vi "TelloDemoExample.vi"(9 "Command":T6, 10 "Tello IP":T5="192.168.1.10") -> (2 "Return":string)   [LabVIEW 2018]
uses:
  Library/Central Controller/TypeDef/TelloCommands.ctl
  Library/Central Controller/TypeDef/TelloIP.ctl
  Library/Central Controller/TypeDef/VideoOutState.ctl
  <vilib>/Platform/TimedLoop/XDataNode/timing_clust.ctl
  <vilib>/Platform/TimedLoop/XDataNode/nitl_modes.ctl
  <vilib>/Platform/TimedLoop/XDataNode/wakeup.ctl
  <vilib>/addons/control/pid/pid.llb/PID (DBL).vi
  <vilib>/Utility/inputDevices.llb/keyboardAcquire.vi
  <vilib>/Utility/inputDevices.llb/closeKeyboard.vi
  <vilib>/platform/TimedLoop/XDataNode/XDataNode.xnode
  Library/Simple UDP Message/Simple UDP Message.lvlib
  <vilib>/Platform/TimedLoop/XDataNode/XDNodeRunTimeDep.lvlib
  <vilib>/addons/control/pid/NI_PID_pid.lvlib
panel:
  out "IterationsPID":i64
  in  "Time switch back to frame from Tello":dbl=0.2 caption="Time Target (s)"
  in  "bkgY":i32=240
  out "VideoState":T1
  out "VideoOut":T2(plugin-control)
  out "Time has Elapsed":bool
  out "TellodetBallFalse":bool
  out "frameFromCam":T2(plugin-control)
  in  "Min Radius (Circle Detection 1) 2":sgl(slide)=9.0 scale=0.0..10.0
  in  "Max Radius (Circle Detection 1) 2":sgl(slide)=100.0 scale=10.0..50.0
  out "Nb Circles2":i32
  out "Circles Data (Circle Detection 1) 2":T3(array[cluster])
  out "Pos. X 2":i32
  in  "Red or Hue Range (Color Threshold 1) 2":cluster{"Lower value":i32, "Upper value":i32}={"Lower value"=20, "Upper value"=40}
  in  "Green or Sat Range (Color Threshold 1) 2":cluster{"Lower value":i32, "Upper value":i32}={"Lower value"=100, "Upper value"=250}
  in  "Blue or Luma or Val or Inten Range (Color Threshold 1) 2":cluster{"Lower value":i32, "Upper value":i32}={"Lower value"=98, "Upper value"=250}
  out "Pos. Y 2":i32
  in  "setpointY":dbl=150.0 format="%#_13g"
  in  "Up/Down PID":T4={"proportional gain (Kc)"=0.30000000000000004, "integral time (Ti, min)"=0.0, "derivative time (Td, min)"=0.001} {"derivative time (Td, min)" format="%.4f"; "integral time (Ti, min)" format="%.4f"; "proportional gain (Kc)" format="%.3f"}
  out "Pos. Y":i32
  in  "Blue or Luma or Val or Inten Range (Color Threshold 1)":cluster{"Lower value":i32, "Upper value":i32}={"Lower value"=98, "Upper value"=250}
  in  "Green or Sat Range (Color Threshold 1)":cluster{"Lower value":i32, "Upper value":i32}={"Lower value"=100, "Upper value"=250}
  in  "Red or Hue Range (Color Threshold 1)":cluster{"Lower value":i32, "Upper value":i32}={"Lower value"=20, "Upper value"=40}
  in  "Yaw PID":T4={"proportional gain (Kc)"=0.233, "integral time (Ti, min)"=0.0, "derivative time (Td, min)"=0.001} {"derivative time (Td, min)" format="%.4f"; "integral time (Ti, min)" format="%.4f"; "proportional gain (Kc)" format="%.3f"}
  out "Pos. X":i32
  in  "followBall":bool
  in  "Ball Detect":bool
  out "Circles Data (Circle Detection 1)":T3(array[cluster])
  out "Nb Circles1":i32
  in  "Max Radius (Circle Detection 1)":sgl(slide)=100.0 scale=10.0..50.0
  in  "Min Radius (Circle Detection 1)":sgl(slide)=9.0 scale=0.0..10.0
  out "frameFromTello":T2(plugin-control)
  out "Stop":bool
  out "RC command String":string
  in  "fly?":bool
  out "tilt l/r, f/b":cluster{dbl[], dbl[]}(graph)
  out "yaw, up/down":cluster{dbl[], dbl[]}(graph)
  out "rc command":string
  out "commands":i32
  out "restart":i32
  out "trials":i32
  in  "Send Cmd":bool
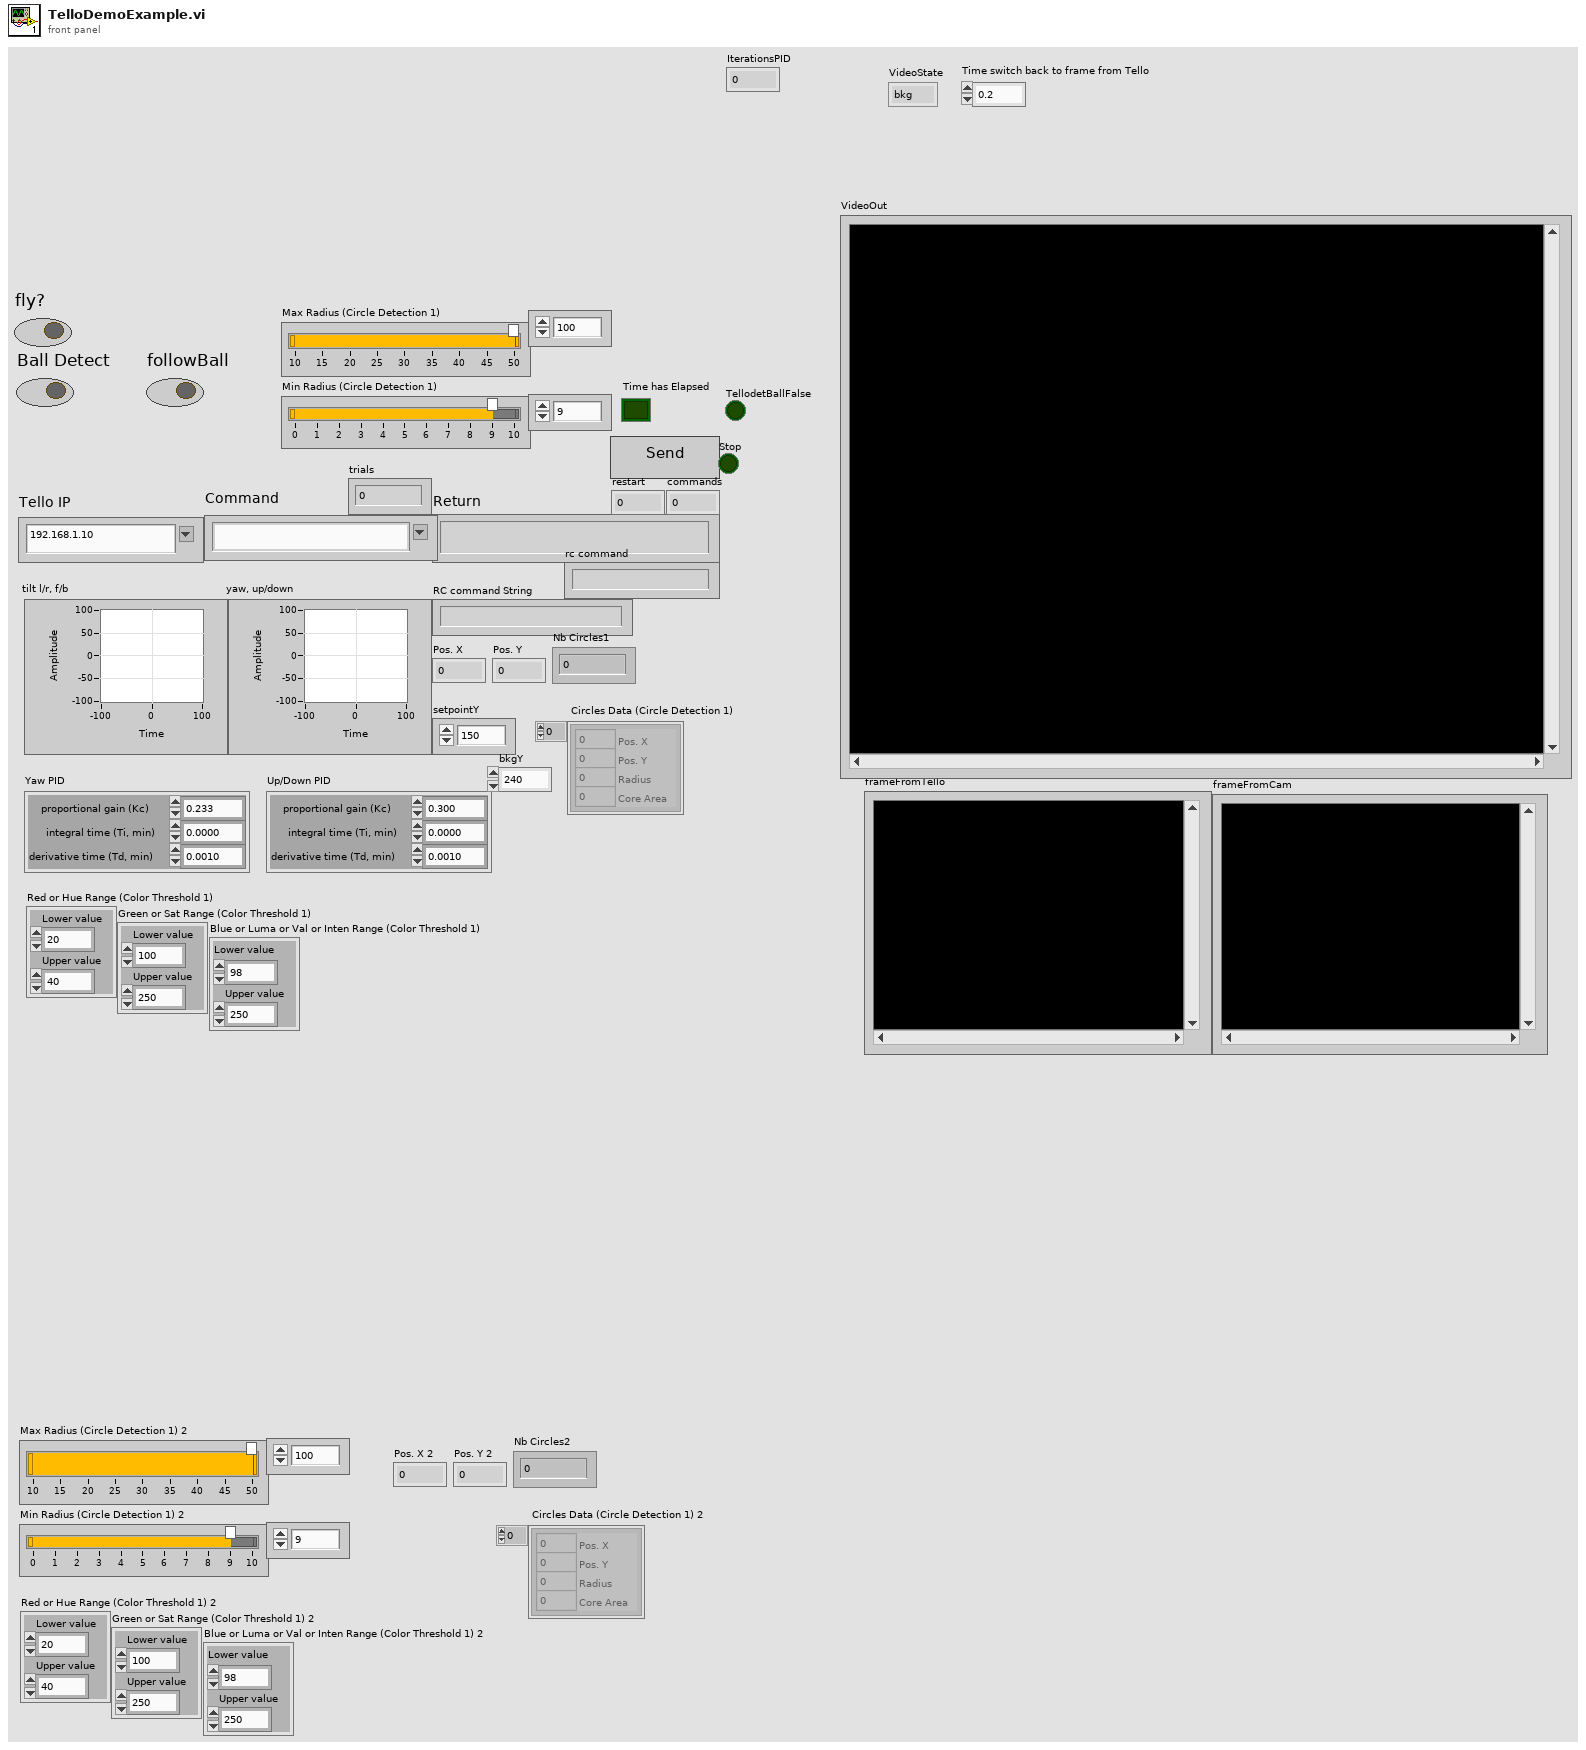
[diagram p1: front panel]
types:
  T1 = typedef "VideoOutState.ctl" = enum16{"bkg", "Tello"}
  T2 = typedef "IMAQ Image.ctl" = refnum<image>
  T3 = cluster{"Pos. X":i32, "Pos. Y":i32, "Radius":i32, "Core Area":i32}[]
  T4 = cluster{"proportional gain (Kc)":dbl, "integral time (Ti, min)":dbl, "derivative time (Td, min)":dbl}
  T5 = typedef "TelloIP.ctl" = string
  T6 = typedef "TelloCommands.ctl" = string
  T7 = typedef "Image Type" = u32
  T8 = typedef "XDNodeRunTimeDep.lvlib/timing_clust.ctl" = cluster{"Expected End [f-1]":u64, "Actual End [f-1]":u64, "Finished Late? [f-1]":bool, "Expected End [i-1]":u64, "Actual End [i-1]":u64, "Finished Late? [i-1]":bool, "Expected Start [i]":u64, "Actual Start [i]":u64, "Expected Start [f]":u64, "Actual Start [f]":u64, "Source Name":string, "Structure Name":string, "Period":i64, "Deadline":i64, "Offset":i64, "Start":i64, "Priority":i32, "Timeout":i32, "Mode":T9, "Wakeup Reason":T10, "Error":errorcluster, "Source Type":string, "Secondary Source Type":string, "Global End Time":u64, "Global Start Time":u64, "Frame Duration":u64, "Iteration Duration":u64, "Assigned CPU":i32, "I/O Scan Engine Mode":u32}
  T9 = typedef "XDNodeRunTimeDep.lvlib/nitl_modes.ctl" = enum32{"No Change", "Process missed periods, maintain original phase", "Discard missed periods, maintain original phase", "Process missed periods, ignore original phase", "Discard missed periods, ignore original phase"}
  T10 = typedef "XDNodeRunTimeDep.lvlib/wakeup.ctl" = enum32{"Normal", "Aborted", "Asynchronous wakeup", "Timing source error", "Timed loop error", "Timeout"}
  T11 = enum16{"0", "1", "2", "3", "4", "5", "6", "7", "8", "9", "A", "B", "C", "D", "E", "F", "G", "H", "I", "J", "K", "L", "M", "N", "O", "P", "Q", "R", "S", "T", "U", "V", "W", "X", "Y", "Z", "F1", "F2", "F3", "F4", "F5", "F6", "F7", "F8", "F9", "F10", "F11", "F12", "F13", "F14", "F15", "ADD", "BACK", "BACKSLASH", "CAPITAL", "COMMA", "DECIMAL", "DELETE", "DIVIDE", "DOWN", "END", "EQUALS", "ESCAPE", "GRAVE (`)", "HOME", "INSERT", "LBRACKET", "LCONTROL", "LEFT", "L ALT", "LSHIFT", "LWIN", "MINUS", "MULTIPLY", "NEXT", "NUMLOCK", "NUMPAD_0", "NUMPAD_1", "NUMPAD_2", "NUMPAD_3", "NUMPAD_4", "NUMPAD_5", "NUMPAD_6", "NUMPAD_7", "NUMPAD_8", "NUMPAD_9", "PAUSE", "PERIOD", "PRIOR (PG UP)", "RBRACKET", "RCONTROL", "RETURN", "RIGHT", "R ALT", "RSHIFT", "RWIN", "SCROLL", "SEMICOLON", "SLASH", "SPACE", "SUBTRACT", "TAB", "UP", "ENTER (num pad)", "' (quote)"}
  T12 = enum16{"0", "1", "2", "3", "4", "5", "6", "7", "8", "9", "A", "B", "C", "D", "E", "F", "G", "H", "I", "J", "K", "L", "M", "N", "O", "P", "Q", "R", "S", "T", "U", "V", "W", "X", "Y", "Z", "F1", "F2", "F3", "F4", "F5", "F6", "F7", "F8", "F9", "F10", "F11", "F12", "F13", "F14", "F15", "ADD", "BACK", "BACKSLASH", "CAPITAL", "COMMA", "DECIMAL", "DELETE", "DIVIDE", "DOWN", "END", "EQUALS", "ESCAPE", "GRAVE (`)", "HOME", "INSERT", "LBRACKET", "LCONTROL", "LEFT", "L ALT", "LSHIFT", "LWIN", "MINUS", "MULTIPLY", "NEXT", "NUMLOCK", "NUMPAD_0", "NUMPAD_1", "NUMPAD_2", "NUMPAD_3", "NUMPAD_4", "NUMPAD_5", "NUMPAD_6", "NUMPAD_7", "NUMPAD_8", "NUMPAD_9", "PAUSE", "PERIOD", "PRIOR (PG UP)", "RBRACKET", "RCONTROL", "RETURN", "RIGHT", "R ALT", "RSHIFT", "RWIN", "SCROLL", "SEMICOLON", "SLASH", "SPACE", "SUBTRACT", "TAB", "UP", "ENTER (num pad)", "' (quote)"}[]
  T13 = cluster{"Left":i32, "Top":i32, "Right":i32, "Bottom":i32}
  T14 = cluster{"Pos. X":i32, "Pos. Y":i32, "Radius":i32, "Core Area":i32}
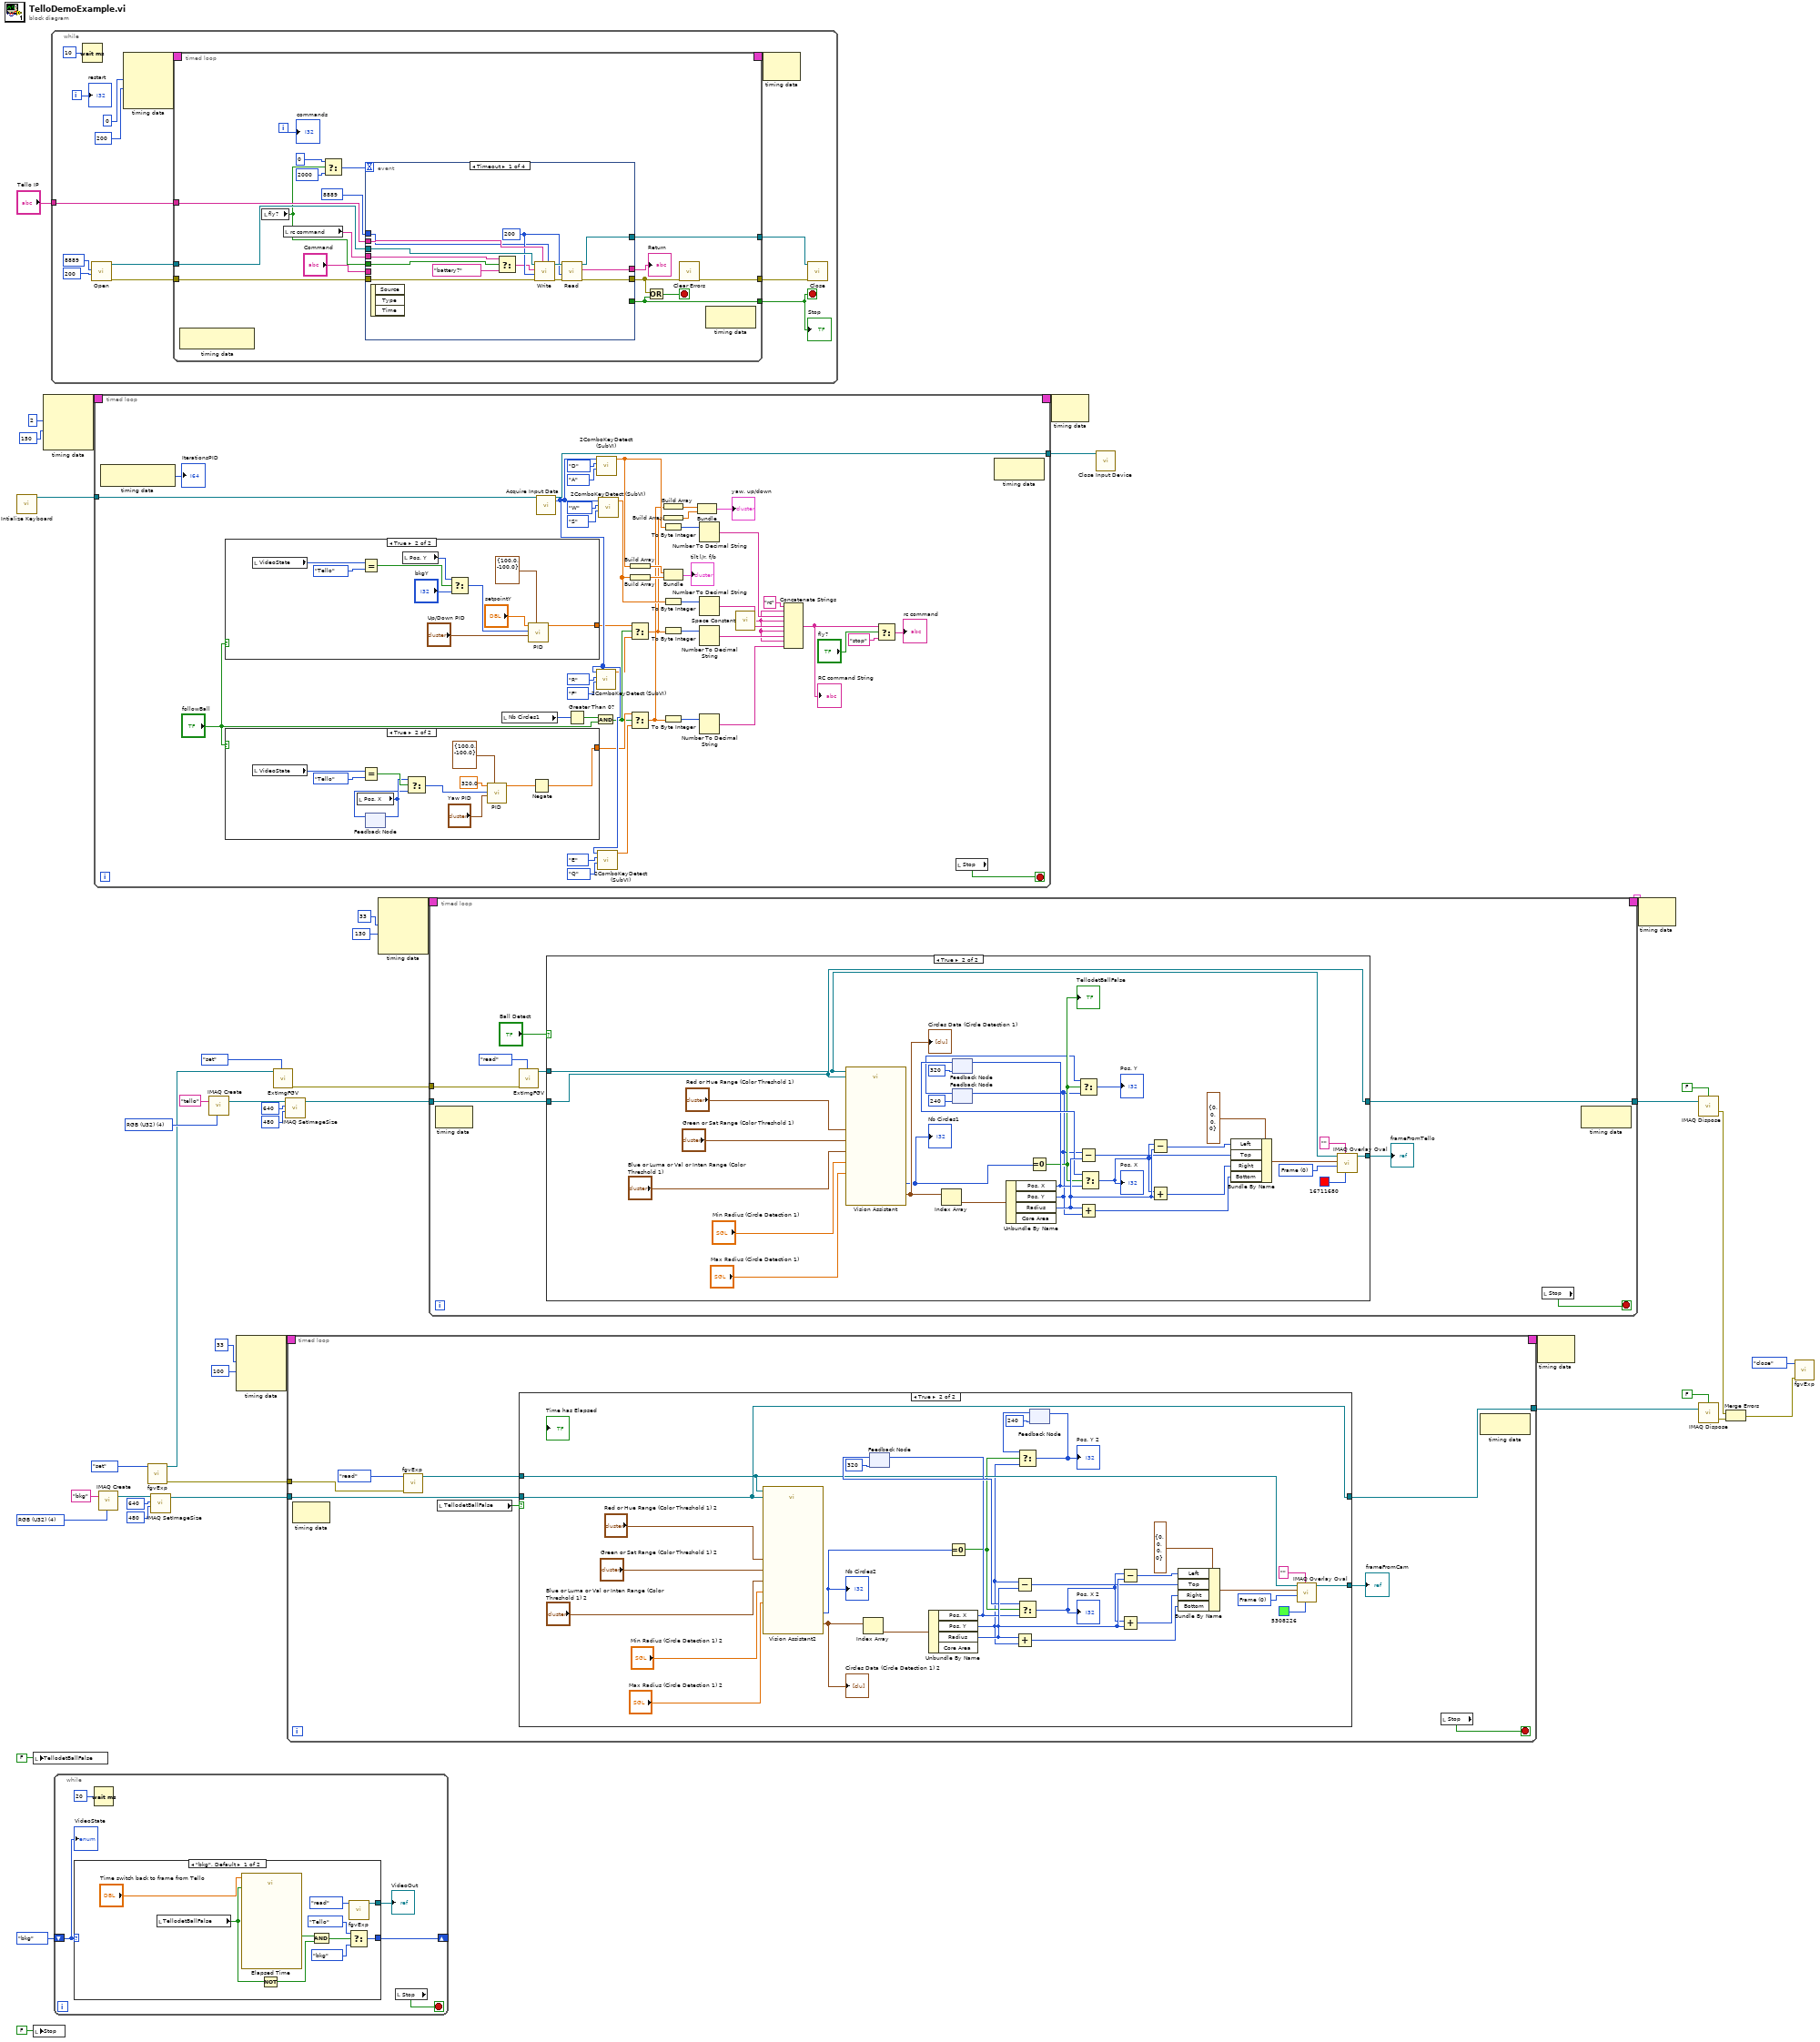
[diagram p0: block diagram]
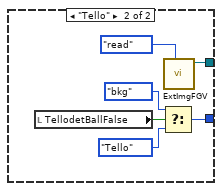
[diagram p2: hidden frame]
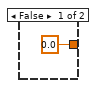
[diagram p5: hidden frame]
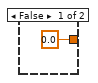
[diagram p6: hidden frame]
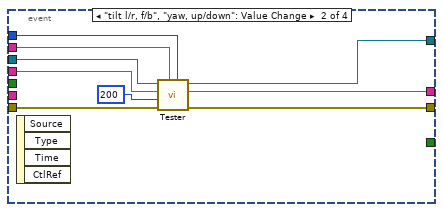
[diagram p7: hidden frame]
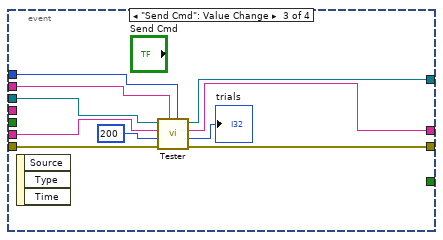
[diagram p8: hidden frame]
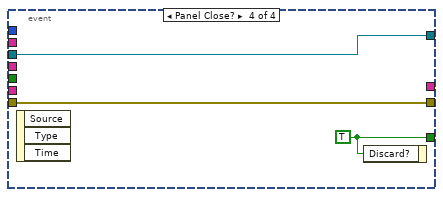
[diagram p9: hidden frame]
diagram:
  w19 = T7 4 items=["Grayscale (U8)", "Grayscale (I16)", "Grayscale (SGL)", "Complex (CSG)", "RGB (U32)", "HSL (U32)", "RGB (U64)", "Grayscale (U16)"] ("Image Type")
  w31 = T7 4 items=["Grayscale (U8)", "Grayscale (I16)", "Grayscale (SGL)", "Complex (CSG)", "RGB (U32)", "HSL (U32)", "RGB (U64)", "Grayscale (U16)"] ("Image Type")
  n1 = call <vilib>:"Intialize Keyboard.vi"() -> ("device ID"=w42:refnum<k1>)  [unwired: 10 in, 1 out]
  n2 = local write "TellodetBallFalse"(FALSE ("1stfail")) -> ()
  n3 = local write "Stop"(FALSE ("Discard?")) -> ()
  n4 = node-c288(i64 2 ("Period"), 150 ("Priority")) -> (w39:T8)  [unwired: 2 in]
  n5 = while {
    tunnel: "Tello IP" -> [w57]
    i -> [w51]
    stop <- w49 stop-if-true
    n6 = Wait (ms)(milliseconds to wait=u32 10) -> ()  [unwired: 1 out]
    n7 = call "Open.vi"("timeout ms (60000)"=200 ("timeout ms (25000)"), "port"=u16 8889) -> ("error out"=w56:errorcluster, "connection ID"=w55:refnum<k16>)  [unwired: 8 in]
    n8 = node-c288(i64 0 ("Period"), 200 ("Priority")) -> (w47:T8)  [unwired: 2 in]
    n9 = timed-loop {
      tunnel: [w70] -> w49
      tunnel: w57 -> [w72]
      tunnel: w56 -> [w68]
      tunnel: w55 -> [w67]
      tunnel: [w66] -> w54
      tunnel: [w65] -> w53
      timing: w47 -> [_]
      timing-out: [_] -> w46
      i -> [w63]
      stop <- w71 stop-if-true
      n10 = node-c288() -> ()  [unwired: 1 in, 1 out]
      n11 = local read "fly?"() -> (w61:bool)
      n12 = local read "rc command"() -> (w62:string)
      n13 = Select(t=0, s=w61, f=2000) -> (s? t:f=w58:i32)
      n14 = event shown="[0] Timeout" {
        selector: _ -> [_ _ _ _]
        dyn-events: _ -> [_ _ _ _]
        timeout: w58 -> [_ _ _ _]
        tunnel: w67 -> [w90 w99 w107 w111]
        tunnel: u16 8889 ("port or service name") -> [w81 w94 w100 _]
        tunnel: w68 -> [w89 w96 w106 w110]
        tunnel: [w86 w95 w109 w110] -> w64
        tunnel: [w84 w98 w108 w111] -> w65
        tunnel: "Command" -> [_ _ w103 _]
        tunnel: [w83 w97 w104 _] -> w74
        tunnel: [_ _ _ w112] -> w70
        tunnel: w72 -> [w88 w93 w105 _]
        tunnel: w62 -> [w79 w92 _ _]
        tunnel: w61 -> [w77 _ _ _]
        event Timeout {
          w82 = 200 ("timeout ms (25000)")
          n15 = event-data() -> ()  [unwired: 1 in, 3 out]
          n16 = Select(t=w79, s=w77, f="battery?" ("data in")) -> (s? t:f=w78:string)
          n17 = call "Write.vi"("port or service name"=w81, "IP"=w88, "error in (no error)"=w89, "timeout ms (25000)"=w82, "data in"=w78, "connection ID"=w90) -> ("error out"=w87:errorcluster, "connection ID"=w85:refnum<k16>)  [unwired: 4 in]
          n18 = call "Read.vi"("error in (no error)"=w87, "timeout ms (25000)"=w82, "connection ID"=w85) -> ("error out"=w86:errorcluster, "data out"=w83:string, "connection ID"=w84:refnum<k16>)  [unwired: 4 in, 2 out]
        }
        event "tilt l/r, f/b", "yaw, up/down": Value Change {
          n19 = event-data() -> ()  [unwired: 1 in, 4 out]
          n20 = call "Tester.vi"("port or service name"=w94, "IP"=w93, "error in (no error)"=w96, "timeout ms (25000)"=200, "Command"=w92, "connection ID"=w99) -> ("error out"=w95:errorcluster, "checker"=w97:string, "connection ID"=w98:refnum<k16>)  [unwired: 2 in, 1 out]
        }
        event "Send Cmd": Value Change {
          n21 = event-data() -> ()  [unwired: 1 in, 3 out]
          n22 = call "Tester.vi"("port or service name"=w100, "IP"=w105, "error in (no error)"=w106, "timeout ms (25000)"=200, "Command"=w103, "connection ID"=w107) -> ("error out"=w109:errorcluster, "iteration"=→"trials":i32, "checker"=w104:string, "connection ID"=w108:refnum<k16>)  [unwired: 2 in]
        }
        event Panel Close? {
          w112 = TRUE ("Discard?")
          n23 = event-data() -> ()  [unwired: 1 in, 3 out]
          n24 = event-data("Discard?"=w112) -> ()  [unwired: 1 in, 1 out]
        }
      }
      "Return" <- w74
      n25 = Or(x=w64, y=w70) -> (x .or. y?=w71:bool)
      n26 = call <vilib>:"Clear Errors.vi"("error in (no error)"=w64) -> ("error out"=w66:errorcluster)  [unwired: 5 in, 1 out]
      n27 = node-c288() -> ()  [unwired: 1 in, 1 out]
      "commands" <- w63
    }
    "Stop" <- w49
    n28 = node-c288(w46) -> ()  [unwired: 1 out]
    n29 = call "Close.vi"("error in (no error)"=w54, "connection ID"=w53) -> ()  [unwired: 9 in, 1 out]
    "restart" <- w51
  }
  n30 = while {
    shift-right: [w119] -> _
    shift-left: VideoOutState."bkg" -> [w121]
    stop <- w118 stop-if-true
    n31 = case shown="\"bkg\", Default" w121 {
      tunnel: [w131 w137] -> w120
      tunnel: [w124 w133] -> w119
      frame "bkg", Default {
        n32 = local read "TellodetBallFalse"() -> (w126:bool)
        n33 = call "Elapsed Time"("Time Target (s)"="Time switch back to frame from Tello", "Reset"=w126) -> ("Time has Elapsed"=w130:bool)  [unwired: 10 in, 7 out]
        n34 = Not(x=w126) -> (.not. x?=w128:bool)
        n35 = And(x=w130, y=w128) -> (x .and. y?=w129:bool)
        n36 = Select(t=VideoOutState."Tello", s=w129, f=VideoOutState."bkg") -> (s? t:f=w124:T1)
        n37 = call "fgvExp.vi"("Enum"=enum16{"set", "read", "close"}."read") -> ("Image Out fgv"=w131:T2)  [unwired: 9 in, 1 out]
      }
      frame "Tello" {
        n38 = local read "TellodetBallFalse"() -> (w136:bool)
        n39 = Select(t=VideoOutState."bkg", s=w136, f=VideoOutState."Tello") -> (s? t:f=w133:T1)
        n40 = call "ExtImgFGV.vi"("Enum"=enum16{"set", "read", "close"}."read") -> ("Image Out"=w137:T2)  [unwired: 9 in, 1 out]
      }
    }
    "VideoOut" <- w120
    n41 = Wait (ms)(milliseconds to wait=u32 20) -> ()  [unwired: 1 out]
    n42 = local read "Stop"() -> (w118:bool)
    "VideoState" <- w121
  }
  n43 = timed-loop {
    tunnel: w42 -> [w183]
    tunnel: [w176] -> w41
    timing: w39 -> [_]
    timing-out: [_] -> w38
    stop <- w152 stop-if-true
    n44 = node-c288() -> (→"IterationsPID":i64)  [unwired: 1 in]
    n45 = case shown="True" "followBall" {
      tunnel: [0.0 ("output") w191] -> w142
      frame False {
      }
      frame True {
        n46 = local read "VideoState"() -> (w189:T1)
        n47 = Equal?(x=w189, y=VideoOutState."Tello") -> (x = y?=w188:bool)
        n48 = local read "Pos. Y"() -> (w187:i32)
        n49 = Select(t=w187, s=w188, f="bkgY") -> (s? t:f=w185:i32)
        n50 = call-poly <vilib>:"PID.vi"("output range"=cluster{"output high":dbl, "output low":dbl} {"output high"=100.0, "output low"=-100.0}, "PID gains"="Up/Down PID", "process variable"=w185, "setpoint"="setpointY") -> ("output"=w191:dbl)  [unwired: 6 in, 1 out]
      }
    }
    n51 = case shown="True" "followBall" {
      tunnel: [0.0 ("output") w202] -> w145
      frame False {
      }
      frame True {
        n52 = local read "VideoState"() -> (w201:T1)
        n53 = local read "Pos. X"() -> (w197:i32)
        n54 = Equal?(x=w201, y=VideoOutState."Tello") -> (x = y?=w199:bool)
        n55 = feedback-in #1(w197) -> ()
        n56 = feedback #1() -> (w196:i32)  [unwired: 1 in]
        n57 = Select(t=w197, s=w199, f=w196) -> (s? t:f=w198:i32)
        n58 = call-poly <vilib>:"PID.vi"("output range"=cluster{"output high":dbl, "output low":dbl} {"output high"=100.0, "output low"=-100.0}, "PID gains"="Yaw PID", "process variable"=w198, "setpoint"=320.0) -> ("output"=w203:dbl)  [unwired: 6 in, 1 out]
        n59 = Negate(x=w203) -> (-x=w202:dbl)
      }
    }
    n60 = local read "Nb Circles1"() -> (w149:i32)
    n61 = call-poly <vilib>:"Acquire Input Data.vi"("device ID"=w183) -> ("device ID"=w176:refnum<k1>, "keys pressed"=w171:T12)  [unwired: 16 in, 1 out]
    n62 = Greater Than 0?(x=w149) -> (x > 0?=w148:bool)
    n63 = call "2ComboKeyDetect (SubVI).vi"("negKey"=T11."F" ("element"), "posKey"=T11."R" ("element"), "keys pressed"=w171) -> ("speedout"=w143:dbl)  [unwired: 8 in]
    n64 = And(x=w148, y="followBall") -> (x .and. y?=w144:bool)
    n65 = call "2ComboKeyDetect (SubVI).vi"("negKey"=T11."A" ("element"), "posKey"=T11."D" ("element"), "keys pressed"=w171) -> ("speedout"=w168:dbl)  [unwired: 8 in]
    n66 = call "2ComboKeyDetect (SubVI).vi"("negKey"=T11."Q" ("element"), "posKey"=T11."E" ("element"), "keys pressed"=w171) -> ("speedout"=w147:dbl)  [unwired: 8 in]
    n67 = call "2ComboKeyDetect (SubVI).vi"("negKey"=T11."S" ("element"), "posKey"=T11."W" ("element"), "keys pressed"=w171) -> ("speedout"=w167:dbl)  [unwired: 8 in]
    n68 = Build Array(w168) -> (w178:dbl[])
    n69 = Build Array(w167) -> (w177:dbl[])
    n70 = Select(t=w142, s=w144, f=w143) -> (s? t:f=w141:dbl)
    n71 = Select(t=w145, s=w144, f=w147) -> (s? t:f=w146:dbl)
    n72 = To Byte Integer(number=w168) -> (8bit integer=w165:i8)
    n73 = To Byte Integer(number=w167) -> (8bit integer=w163:i8)
    n74 = To Byte Integer(number=w141) -> (8bit integer=w161:i8)
    n75 = To Byte Integer(number=w146) -> (8bit integer=w157:i8)
    n76 = Build Array(w146) -> (w170:dbl[])
    n77 = Build Array(w141) -> (w169:dbl[])
    n78 = Bundle(w178, w177) -> (→"tilt l/r, f/b":cluster{dbl[], dbl[]})  [unwired: 1 in]
    n79 = Bundle(w170, w169) -> (→"yaw, up/down":cluster{dbl[], dbl[]})  [unwired: 1 in]
    n80 = Number To Decimal String(number=w165) -> (decimal integer string=w164:string)  [unwired: 1 in]
    n81 = Number To Decimal String(number=w163) -> (decimal integer string=w162:string)  [unwired: 1 in]
    n82 = Number To Decimal String(number=w161) -> (decimal integer string=w160:string)  [unwired: 1 in]
    n83 = Number To Decimal String(number=w157) -> (decimal integer string=w158:string)  [unwired: 1 in]
    n84 = call <vilib>:"Space Constant.vi"() -> ("String"=w159:string)
    n85 = Concatenate Strings("rc" ("string"), w159, w164, w159, w162, w159, w160, w159, w158) -> (w155:string)
    "RC command String" <- w155
    n86 = Select(t=w155, s="fly?", f="stop") -> (s? t:f=→"rc command":string)
    n87 = local read "Stop"() -> (w152:bool)
    n88 = node-c288() -> ()  [unwired: 1 in, 1 out]
  }
  n89 = call "IMAQ Create"("Image Name"="bkg", "Image Type"=w19) -> ("New Image"=w22:T2)  [unwired: 3 in, 1 out]
  n90 = call "fgvExp.vi"("Enum"=enum16{"set", "read", "close"}."set") -> ("error out"=w4:errorcluster, "Image Out fgv"=w1:T2)  [unwired: 9 in]
  n91 = call "IMAQ SetImageSize"("Y Resolution"=480, "X Resolution"=640, "Image"=w22) -> ("Image Out"=w17:T2)  [unwired: 2 in, 1 out]
  n92 = call "IMAQ Create"("Image Name"="tello", "Image Type"=w31) -> ("New Image"=w27:T2)  [unwired: 3 in, 1 out]
  n93 = node-c288(i64 33 ("Period"), 100 ("Priority")) -> (w25:T8)  [unwired: 2 in]
  n94 = call "ExtImgFGV.vi"("Enum"=enum16{"set", "read", "close"}."set", "Image In"=w1) -> ("error out"=w2:errorcluster)  [unwired: 8 in, 1 out]
  n95 = call "IMAQ SetImageSize"("Y Resolution"=480, "X Resolution"=640, "Image"=w27) -> ("Image Out"=w28:T2)  [unwired: 2 in, 1 out]
  n96 = timed-loop {
    timing: w25 -> [_]
    timing-out: [_] -> w24
    tunnel: w17 -> [w216]
    tunnel: [w214] -> w14
    tunnel: w4 -> [w210]
    stop <- w217 stop-if-true
    n97 = node-c288() -> ()  [unwired: 1 in, 1 out]
    n98 = call "fgvExp.vi"("error in"=w210, "Enum"=enum16{"set", "read", "close"}."read") -> ("Image Out fgv"=w211:T2)  [unwired: 8 in, 1 out]
    n99 = local read "TellodetBallFalse"() -> (w213:bool)
    n100 = case shown="True" w213 {
      tunnel: w216 -> [w219 w234]
      tunnel: [w218 w235] -> w215
      tunnel: [w219 w234] -> w214
      tunnel: w211 -> [w218 w225]
      frame False {
      }
      frame True {
        w247 = u32 0 items=["Frame", "Fill"] ("Drawing Mode (Frame)")
        n101 = call "Vision Assistant2"("Image In"=w225, "Image Dst"=w234, "Red or Hue Range (Color Threshold 1)"="Red or Hue Range (Color Threshold 1) 2", "Min Radius (Circle Detection 1)"="Min Radius (Circle Detection 1) 2", "Max Radius (Circle Detection 1)"="Max Radius (Circle Detection 1) 2", "Green or Sat Range (Color Threshold 1)"="Green or Sat Range (Color Threshold 1) 2", "Blue or Luma or Val or Inten Range (Color Threshold 1)"="Blue or Luma or Val or Inten Range (Color Threshold 1) 2") -> ("Nb Circles (Circle Detection 1)"=w230:i32, "Circles Data (Circle Detection 1)"=w237:T3)  [unwired: 17 in, 2 out]
        "Nb Circles2" <- w230
        "Circles Data (Circle Detection 1) 2" <- w237
        n102 = Index Array(array=w237) -> (element=w246:T14)  [unwired: 1 in]
        n103 = feedback #2(320 ("Pos. X")) -> (w229:i32)
        n104 = Unbundle By Name(w246) -> ("Pos. X"=w228:i32, "Pos. Y"=w223:i32, "Radius"=w242:i32)  [unwired: 1 out]
        n105 = feedback-in #2(w228) -> ()
        n106 = Equal To 0?(x=w230) -> (x = 0?=w224:bool)
        n107 = Subtract(x=w223, y=w242) -> (x-y=w241:i32)
        n108 = Add(x=w242, y=w223) -> (x+y=w243:i32)
        n109 = Select(t=w229, s=w224, f=w228) -> (s? t:f=w227:i32)
        "Pos. X 2" <- w227
        n110 = feedback #3(240 ("Pos. Y")) -> (w222:i32)
        n111 = Select(t=w222, s=w224, f=w223) -> (s? t:f=w220:i32)
        "Pos. Y 2" <- w220
        n112 = feedback-in #3(w220) -> ()
        n113 = Subtract(x=w227, y=w242) -> (x-y=w245:i32)
        n114 = Add(x=w227, y=w242) -> (x+y=w244:i32)
        n115 = Bundle By Name(cluster=T13 {"Left"=0, "Top"=0, "Right"=0, "Bottom"=0} ("Bounding Rectangle"), "Left"=w245, "Top"=w241, "Right"=w244, "Bottom"=w243) -> (w240:T13)
        n116 = call "IMAQ Overlay Oval"("Color"=u32 5308226, "Group"="", "Drawing Mode (Frame)"=w247, "Bounding Rectangle"=w240, "Image"=w225) -> ("Image Out"=w235:T2)  [unwired: 5 in, 1 out]
      }
    }
    "frameFromCam" <- w215
    n117 = local read "Stop"() -> (w217:bool)
    n118 = node-c288() -> ()  [unwired: 1 in, 1 out]
  }
  n119 = node-c288(i64 33 ("Period"), 130 ("Priority")) -> (w36:T8)  [unwired: 2 in]
  n120 = timed-loop {
    timing: w36 -> [_]
    timing-out: [_] -> w35
    tunnel: w28 -> [w258]
    tunnel: [w253] -> w26
    tunnel: w2 -> [w252]
    stop <- w259 stop-if-true
    n121 = node-c288() -> ()  [unwired: 1 in, 1 out]
    n122 = call "ExtImgFGV.vi"("Enum"=enum16{"set", "read", "close"}."read", "error in"=w252) -> ("Image Out"=w255:T2)  [unwired: 8 in, 1 out]
    n123 = case shown="True" "Ball Detect" {
      tunnel: w258 -> [w260 w276]
      tunnel: [w261 w277] -> w254
      tunnel: w255 -> [w261 w267]
      tunnel: [w260 w276] -> w253
      frame False {
      }
      frame True {
        w289 = u32 0 items=["Frame", "Fill"] ("Drawing Mode (Frame)")
        n124 = call "Vision Assistant"("Image In"=w267, "Image Dst"=w276, "Red or Hue Range (Color Threshold 1)"="Red or Hue Range (Color Threshold 1)", "Min Radius (Circle Detection 1)"="Min Radius (Circle Detection 1)", "Max Radius (Circle Detection 1)"="Max Radius (Circle Detection 1)", "Green or Sat Range (Color Threshold 1)"="Green or Sat Range (Color Threshold 1)", "Blue or Luma or Val or Inten Range (Color Threshold 1)"="Blue or Luma or Val or Inten Range (Color Threshold 1)") -> ("Nb Circles (Circle Detection 1)"=w272:i32, "Circles Data (Circle Detection 1)"=w279:T3)  [unwired: 17 in, 2 out]
        "Nb Circles1" <- w272
        "Circles Data (Circle Detection 1)" <- w279
        n125 = Index Array(array=w279) -> (element=w288:T14)  [unwired: 1 in]
        n126 = feedback #4(320 ("Pos. X")) -> (w271:i32)
        n127 = feedback #5(240 ("Pos. Y")) -> (w263:i32)
        n128 = Unbundle By Name(w288) -> ("Pos. X"=w270:i32, "Pos. Y"=w264:i32, "Radius"=w284:i32)  [unwired: 1 out]
        n129 = feedback-in #4(w270) -> ()
        n130 = feedback-in #5(w264) -> ()
        n131 = Equal To 0?(x=w272) -> (x = 0?=w265:bool)
        "TellodetBallFalse" <- w265
        n132 = Select(t=w263, s=w265, f=w264) -> (s? t:f=→"Pos. Y":i32)
        n133 = Subtract(x=w264, y=w284) -> (x-y=w283:i32)
        n134 = Add(x=w284, y=w264) -> (x+y=w285:i32)
        n135 = Select(t=w271, s=w265, f=w270) -> (s? t:f=w269:i32)
        "Pos. X" <- w269
        n136 = Subtract(x=w269, y=w284) -> (x-y=w287:i32)
        n137 = Add(x=w269, y=w284) -> (x+y=w286:i32)
        n138 = Bundle By Name(cluster=T13 {"Left"=0, "Top"=0, "Right"=0, "Bottom"=0} ("Bounding Rectangle"), "Left"=w287, "Top"=w283, "Right"=w286, "Bottom"=w285) -> (w282:T13)
        n139 = call "IMAQ Overlay Oval"("Color"=u32 16711680, "Group"="", "Drawing Mode (Frame)"=w289, "Bounding Rectangle"=w282, "Image"=w267) -> ("Image Out"=w277:T2)  [unwired: 5 in, 1 out]
      }
    }
    "frameFromTello" <- w254
    n140 = local read "Stop"() -> (w259:bool)
    n141 = node-c288() -> ()  [unwired: 1 in, 1 out]
  }
  n142 = node-c288(w38) -> ()  [unwired: 1 out]
  n143 = call-poly <vilib>:"Close Input Device.vi"("device ID"=w41) -> ()  [unwired: 9 in, 1 out]
  n144 = node-c288(w24) -> ()  [unwired: 1 out]
  n145 = node-c288(w35) -> ()  [unwired: 1 out]
  n146 = call "IMAQ Dispose"("All Images? (No)"=FALSE, "Image"=w26) -> ("error out"=w12:errorcluster)  [unwired: 4 in]
  n147 = call "IMAQ Dispose"("All Images? (No)"=FALSE, "Image"=w14) -> ("error out"=w13:errorcluster)  [unwired: 4 in]
  n148 = Merge Errors(w12, w13) -> (w11:errorcluster)
  n149 = call "fgvExp.vi"("error in"=w11, "Enum"=enum16{"set", "read", "close"}."close") -> ()  [unwired: 8 in, 2 out]
